vi "EngineTagsUI.vi"() -> ()   [LabVIEW 2013, in "PL Framework Configuration Tool.lvlib" / "EngineTags.lvclass"]
uses:
  EngineTags.lvclass
  <vilib>/NI/Configuration Framework/Node/NodeRef.ctl
  <vilib>/NI/Configuration Framework/Node/NISE_CEF_Node.lvclass
  <vilib>/NI/AMC/Message Queue.ctl
  <vilib>/NI/AMC/Message.ctl
  <vilib>/NI/Tools/Keyed Array/KeyedArray.ctl
  <vilib>/NI/Configuration Framework/Node/UserEventRef.ctl
  <vilib>/NI/Configuration Framework/Controls/EventCluster.ctl
  <vilib>/NI/Tag Bus/tag/Data Type.ctl
  <vilib>/NI/Configuration Framework/Node/RefreshUIEvent.ctl
  <vilib>/NI/Configuration Framework/Node/CacheState.ctl
  <vilib>/NI/Configuration Framework/Node/StopEvent.ctl
  <vilib>/NI/Configuration Framework/Node/NodeChangeEvent.ctl
  additional filter.ctl
  <vilib>/Utility/miscctls.llb/LVPositionTypeDef.ctl
  <vilib>/NI/Module Execution Interface/Engine Configuration/engine configuration.lvclass/engine configuration.ctl
  <vilib>/NI/Tag Bus/tag/tag descriptor.lvclass/tag descriptor.ctl
  <vilib>/NI/Tag Bus/tag/read tag name.vi
  <vilib>/NI/Tag Bus/tag/read data type.vi
  <vilib>/NI/Tag Bus/tag/read raw default value.vi
  <vilib>/NI/Tag Bus/tag/read metadata.vi
  <vilib>/NI/Module Execution Interface/Engine Configuration/engine configuration.lvclass
  Engine Parent/Engine Parent Editor Node.lvclass
  <vilib>/NI/Tag Bus/tag/tag descriptor.lvclass
  <vilib>/NI/Tools/Keyed Array/Tools_KeyedArray.lvlib
  <vilib>/NI/AMC/AMC.lvlib
  <vilib>/NI/Configuration Framework/NISE_CEF_TreeControl.lvlib
panel:
  in  "more filters":T1
  in  "Remove Button":bool
  in  "node change":T2
  in  "stop event":T3
  in  "cache state":T4
  in  "refresh UI":T5
  in  "Filter":string
  in  "export to csv":bool
  in  "open csv":bool
  in  "open cvtv3 taglist":bool
  in  "load CVT1 file":bool
  in  "Create Tag":bool
  in  "data type":T6
  in  "Table":string[][](table)
  in  "user event":T7
  in  "main queue":T8
  in  "node ref":T9
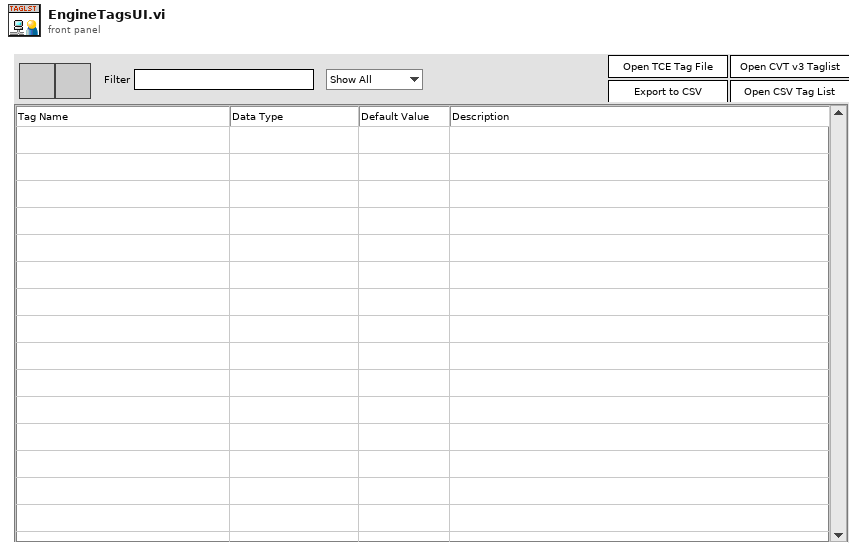
[diagram p1: front panel]
types:
  T1 = typedef "PL Framework Configuration Tool.lvlib/EngineTags.lvclass/additional filter.ctl" = enum16{"Show All", "Show Unmapped"}
  T2 = typedef "NISE_CEF_Node.lvclass/NodeChangeEvent.ctl" = refnum<user-event>
  T3 = typedef "NISE_CEF_Node.lvclass/StopEvent.ctl" = refnum<user-event>
  T4 = typedef "NISE_CEF_Node.lvclass/CacheState.ctl" = refnum<user-event>
  T5 = typedef "NISE_CEF_Node.lvclass/RefreshUIEvent.ctl" = refnum<user-event>
  T6 = typedef "tag bus.lvlib/tag descriptor.lvclass/Data Type.ctl" = enum16{"Double", "Single", "I64", "I32", "I16", "I8", "U64", "U32", "U16", "U8", "Boolean", "String", "Array of Double", "Array of Single", "Array of I64", "Array of I32", "Array of I16", "Array of I8", "Array of U64", "Array of U32", "Array of U16", "Array of U8", "Array of Boolean", "Array of String"}
  T7 = typedef "NISE_CEF_Node.lvclass/UserEventRef.ctl" = refnum<user-event>
  T8 = typedef "AMC.lvlib/Message Queue.ctl" = refnum<queue>
  T9 = typedef "NISE_CEF_Node.lvclass/NodeRef.ctl" = refnum<data-value>
  T10 = typedef "LVPositionTypeDef.ctl" = cluster{"Left":i32, "Top":i32}
  T11 = enum16{"open", "replace", "create", "open or create", "replace or create", "replace or create with confirmation"}
  T12 = typedef "LVPoint32TypeDef.ctl" = cluster{"Horizontal":i32, "Vertical":i32}
  T13 = typedef "LVRowAndColumnTypeDef.ctl" = cluster{"Row":i32, "Column":i32}
  T14 = typedef "LVBoundsTypeDef.ctl" = cluster{"Width":u32, "Height":u32}
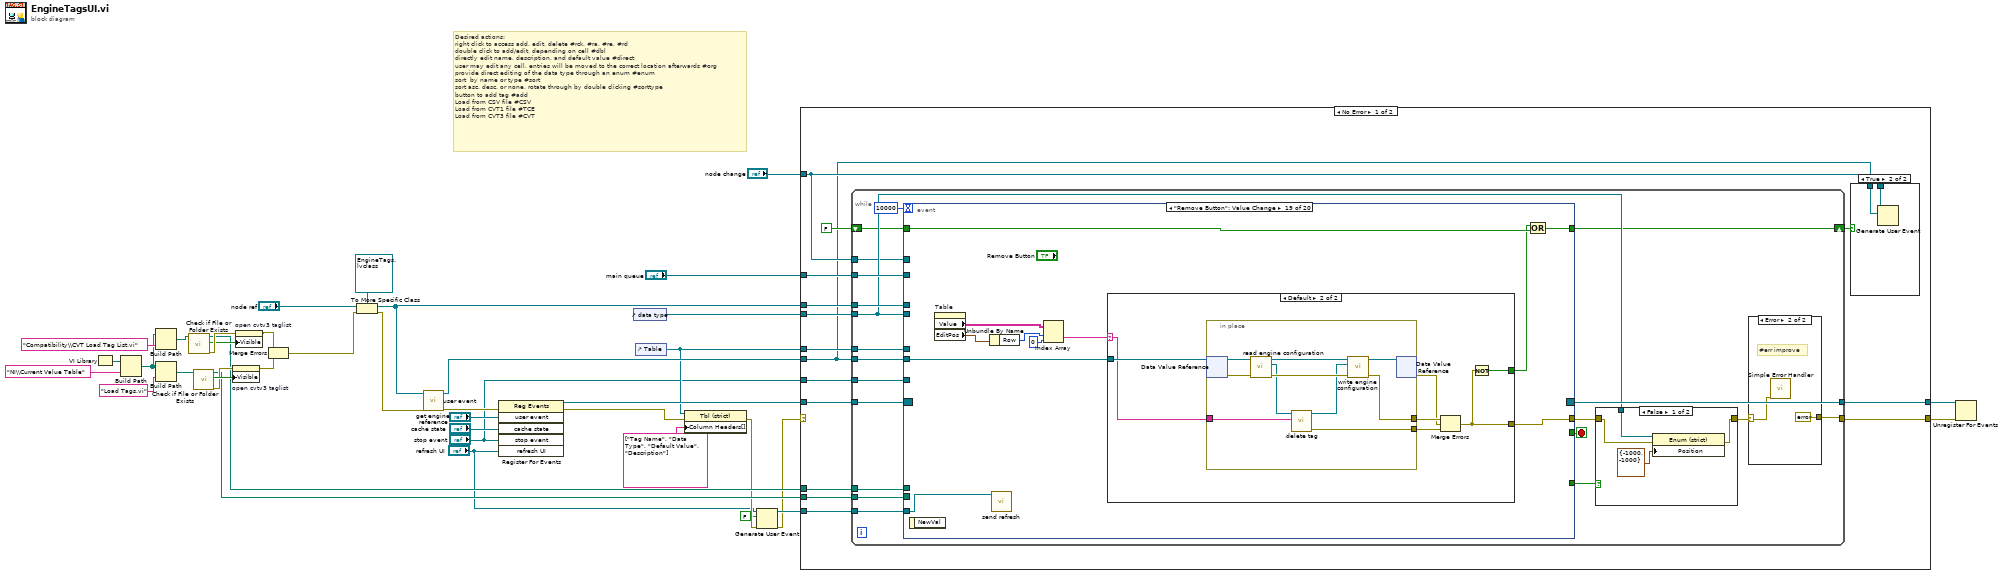
[diagram p0: block diagram]
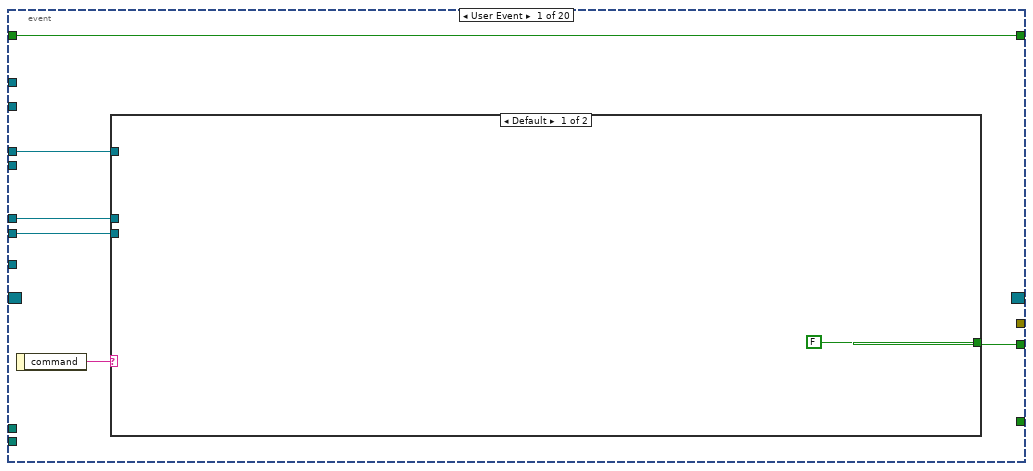
[diagram p5: hidden frame]
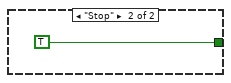
[diagram p6: hidden frame]
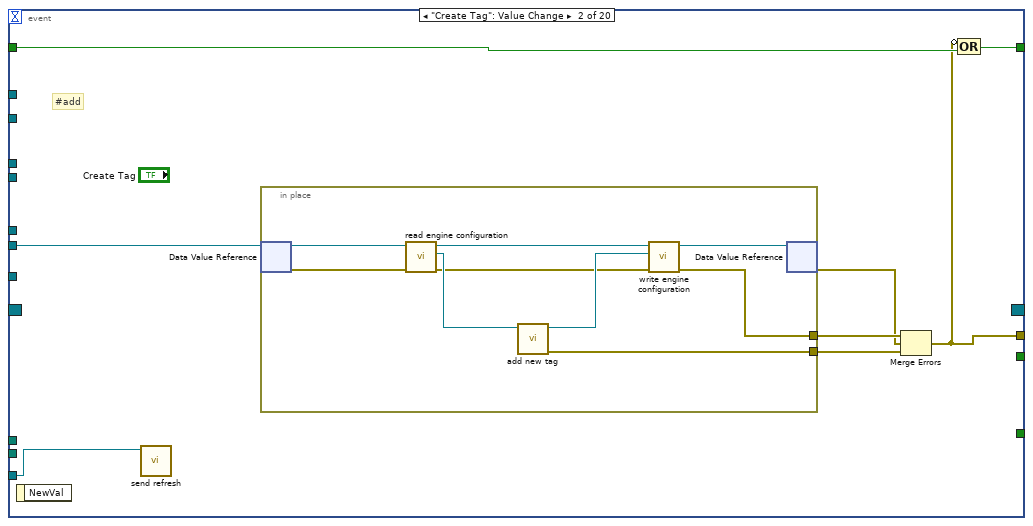
[diagram p7: hidden frame]
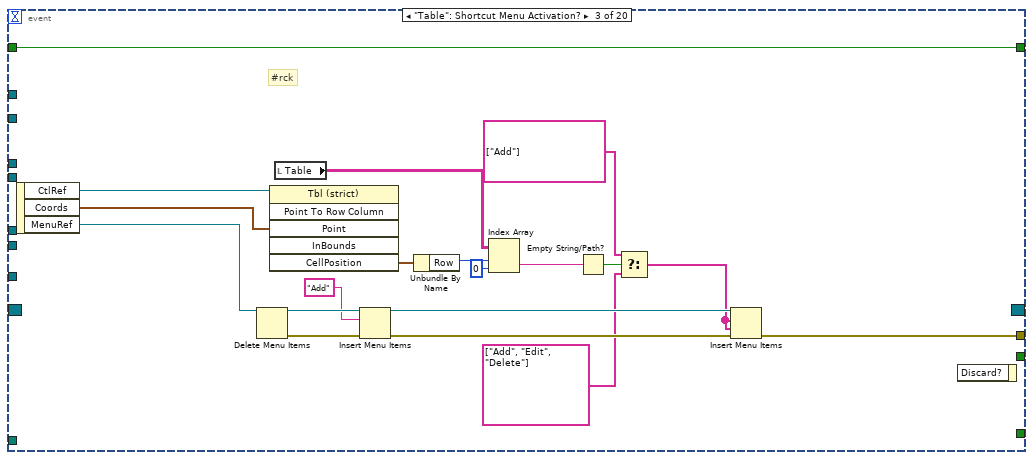
[diagram p8: hidden frame]
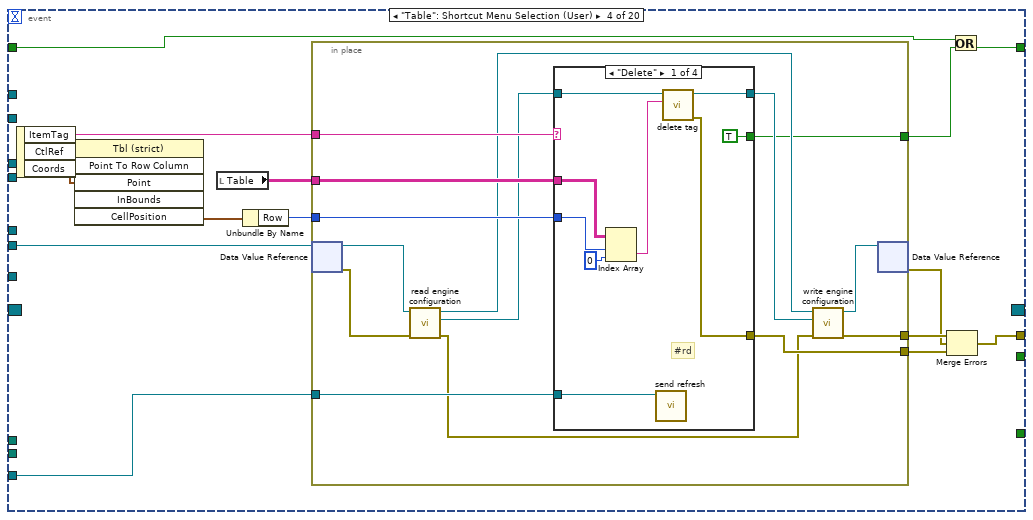
[diagram p9: hidden frame]
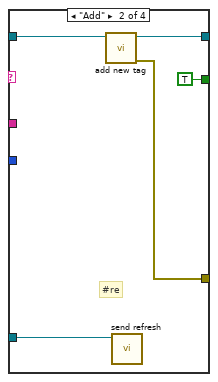
[diagram p10: hidden frame]
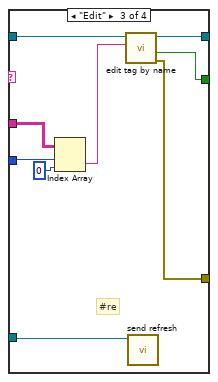
[diagram p11: hidden frame]
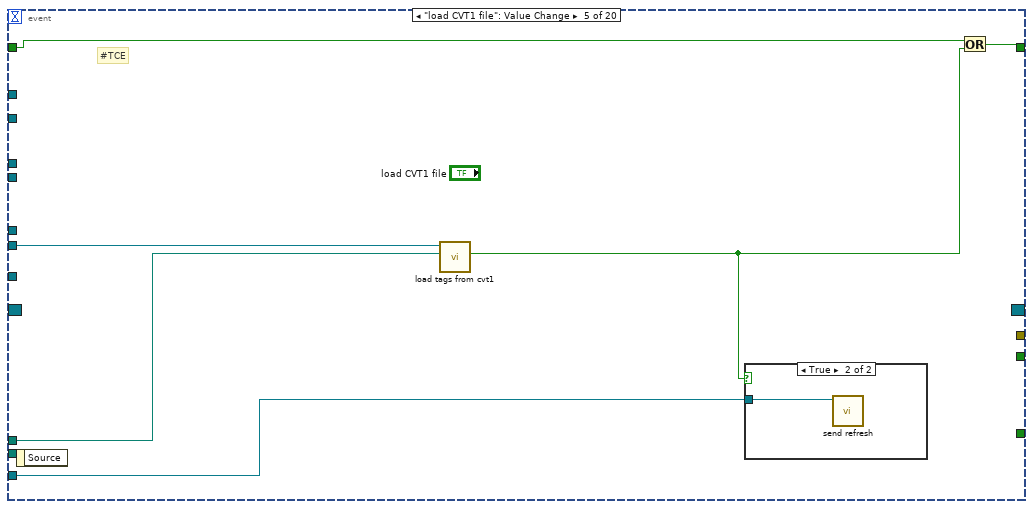
[diagram p13: hidden frame]
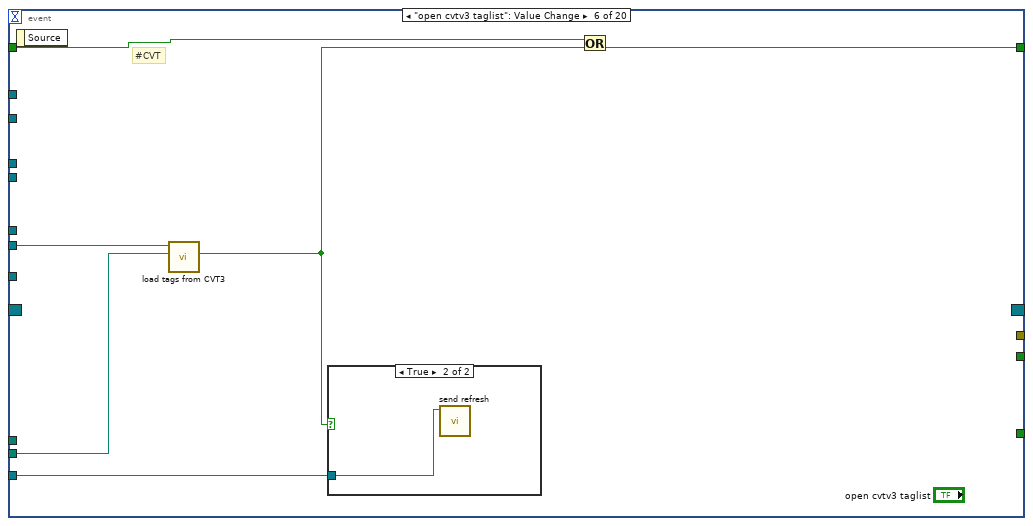
[diagram p15: hidden frame]
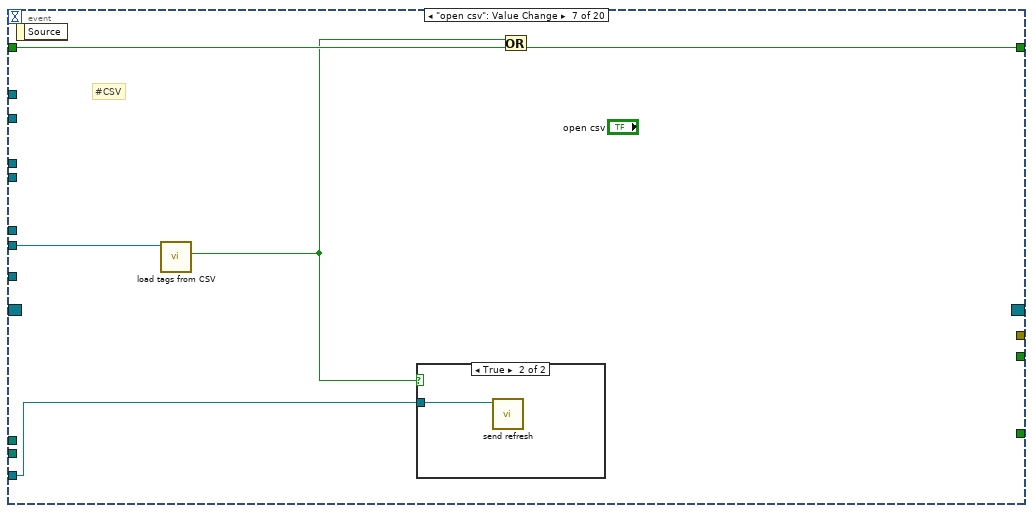
[diagram p17: hidden frame]
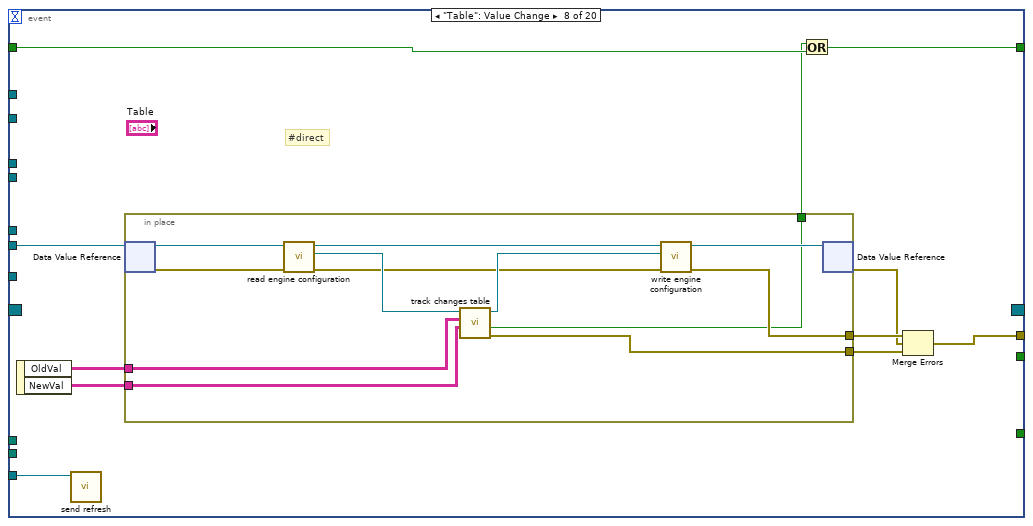
[diagram p19: hidden frame]
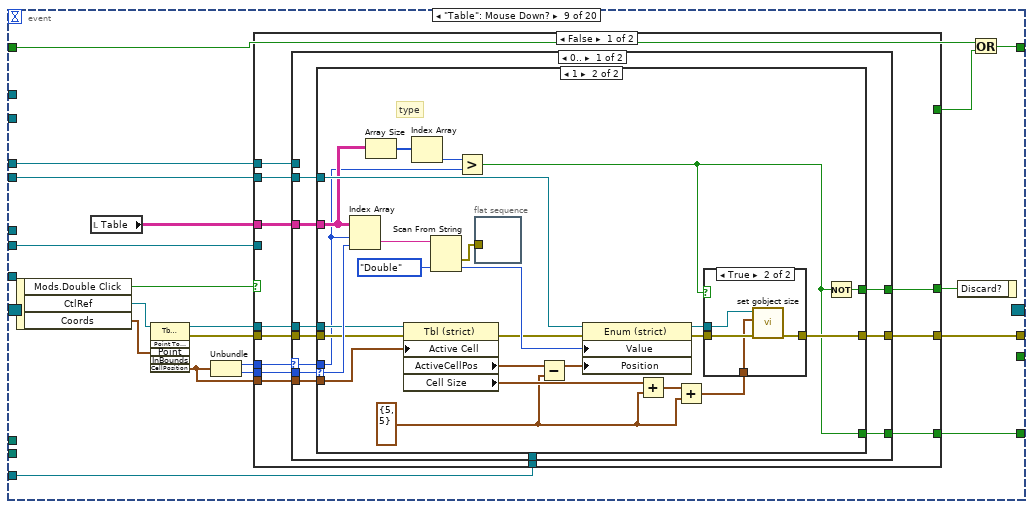
[diagram p20: hidden frame]
diagram:
  # "Desired actions:\nright click to access add, edit, delete #rck, #ra, #re, #rd\ndouble click to add/edit, depending on cell #dbl\ndirectly edit name, description, and default value #direct\nuser may edit any cell, entries will be moved to the correct location afterwards #org\nprovide direct editing of the data type through an enum #enum\nsort  by name or type #sort\nsort asc, desc, or none, rotate through by double clicking #sorttype\nbutton to add tag #add\nLoad from CSV file #CSV\nLoad from CVT1 file #TCE\nLoad from CVT3 file #CVT"
  n1 = VI Library() -> (path=w34:path)
  n2 = Build Path(base path=w34, name or relative path="NI\\Current Value Table") -> (appended path=w30:path)
  n3 = Build Path(base path=w30, name or relative path="Compatibility\\CVT Load Tag List.vi") -> (appended path=w23:path)
  n4 = Build Path(base path=w30, name or relative path="Load Tags.vi") -> (appended path=w21:path)
  n5 = call <vilib>:"Check if File or Folder Exists.vi"("path"=w23) -> ("error out"=w27:errorcluster, "file or folder exists?"=w26:bool, "dup path"=w22:path)  [unwired: 8 in]
  n6 = call <vilib>:"Check if File or Folder Exists.vi"("path"=w21) -> ("error out"=w28:errorcluster, "file or folder exists?"=w29:bool, "dup path"=w20:path)  [unwired: 8 in]
  n7 = property on="open cvtv3 taglist" class="Bool"(error in=w28, "Visible"=w29) -> (error out=w25:errorcluster)  [unwired: 1 in, 1 out]
  n8 = property on="open cvtv3 taglist" class="Bool"(error in=w27, "Visible"=w26) -> (error out=w24:errorcluster)  [unwired: 1 in, 1 out]
  n9 = Merge Errors(w24, w25) -> (w19:errorcluster)
  n10 = To More Specific Class(target class=refnum<data-value> refnum ("data value reference"), reference="node ref", error in=w19) -> (specific class reference=w18:refnum<data-value>, error out=w6:errorcluster)
  n11 = call "get engine reference.vi"("error in"=w6, "enginetags"=w18) -> ("error out"=w15:errorcluster, "engine reference"=w14:refnum<data-value>)  [unwired: 8 in]
  n12 = register-events(error in=w15, "user event", "cache state", "stop event", "refresh UI") -> (reference out=w38:refnum<event-registration>, error out=w35:errorcluster)  [unwired: 1 in]
  n13 = control-ref of="data type"() -> (w16:refnum<vi>)
  n14 = control-ref of="Table"() -> (w13:refnum<vi>)
  n15 = property on="Property Node" class="Tbl (strict)"(reference=w13, error in=w35, "Column Headers[]"=string[] ["Tag Name", "Data Type", "Default Value", "Description"] ("Column Header Strings[]")) -> (error out=w9:errorcluster)  [unwired: 1 out]
  n16 = Generate User Event(user event="refresh UI", event data cluster=FALSE ("event data"), error in=w9) -> (user event out=w10:T5, error out=w8:errorcluster)  [unwired: 1 in]
  n17 = case shown="No Error" w8 {
    selector: w8 -> [_ w514]
    tunnel: "main queue" -> [w54 _]
    tunnel: w38 -> [w53 w515]
    tunnel: [w52 w515] -> w37
    tunnel: [w51 w514] -> w36
    tunnel: w22 -> [w50 _]
    tunnel: w20 -> [w49 _]
    tunnel: w18 -> [w48 _]
    tunnel: w16 -> [w47 _]
    tunnel: w14 -> [w41 _]
    tunnel: w13 -> [w46 _]
    tunnel: w10 -> [w45 _]
    tunnel: "node change" -> [w42 _]
    tunnel: "stop event" -> [w40 _]
    frame No Error {
      n18 = while {
        tunnel: w48 -> [w68]
        tunnel: w54 -> [w76]
        tunnel: w53 -> [w75]
        tunnel: [w74] -> w52
        tunnel: w49 -> [w72]
        tunnel: w50 -> [w71]
        tunnel: w47 -> [w63]
        tunnel: w41 -> [w69]
        tunnel: w46 -> [w67]
        tunnel: w45 -> [w62]
        tunnel: [w70] -> w51
        shift-right: [w58] -> w43
        shift-left: FALSE -> [w59]
        tunnel: w42 -> [w61]
        tunnel: w40 -> [w57]
        stop <- w73 stop-if-true
        n19 = event shown="[18] \"Remove Button\": Value Change" {
          selector: w75 -> [_ _ _ _ _ _ _ _ _ _ _ _ _ _ _ _ w455 _ _ _]
          dyn-events: [_ _ _ _ _ _ _ _ _ _ _ _ _ _ _ _ _ _ _ _] -> w74
          timeout: 10000 -> [_ _ _ _ _ _ _ _ _ _ _ _ _ _ _ _ _ _ _ _]
          tunnel: w68 -> [w87 _ _ _ _ _ _ _ w237 _ _ _ _ _ _ _ w464 _ _ _]
          tunnel: w76 -> [_ _ _ _ _ _ _ _ _ _ _ _ _ _ _ _ _ _ _ _]
          tunnel: [w89 _ _ _ _ _ _ _ _ _ _ _ _ _ _ TRUE FALSE _ _ _] -> w73
          tunnel: w72 -> [_ _ _ _ _ w194 _ _ _ _ _ _ _ _ _ _ _ _ _ _]
          tunnel: w71 -> [_ _ _ _ w187 _ _ _ _ _ _ _ _ _ _ _ _ _ _ _]
          tunnel: [_ w93 w117 w134 _ _ _ w208 w239 w350 w400 w407 _ w440 _ _ w467 _ w488 w510] -> w64
          tunnel: w63 -> [_ _ _ _ _ _ _ _ w233 w369 _ _ _ _ _ _ _ _ _ _]
          tunnel: w69 -> [w90 w99 _ w135 w185 w192 w199 w209 w228 w351 _ w404 _ _ _ _ w466 w475 w492 _]
          tunnel: w67 -> [w86 _ _ _ _ _ _ _ _ w370 _ _ _ _ _ _ w463 _ _ _]
          tunnel: [_ _ _ _ _ _ _ _ w230 _ _ _ _ _ _ _ _ _ _ _] -> w66
          tunnel: w62 -> [_ w95 _ w136 w186 w193 w200 w202 w229 w347 _ _ w437 _ _ _ _ _ w490 w512]
          tunnel: w61 -> [_ _ _ _ _ _ _ _ _ _ _ _ _ _ _ _ _ w476 _ _]
          tunnel: w59 -> [w85 w96 w110 w131 w184 w191 w198 w205 w227 _ w399 w402 w438 w439 w443 w448 w453 w477 w491 w513]
          tunnel: [w85 w94 w110 w130 w183 w190 w197 w204 w226 TRUE w399 w402 w438 w439 w443 w448 w452 w474 w489 w513] -> w58
          tunnel: w57 -> [_ _ _ _ _ _ _ _ _ _ w398 _ _ _ _ _ _ _ _ _]
          event User Event {
            n20 = event-data() -> ("command"=w88:string)  [unwired: 1 in]
            n21 = case shown="Default" w88 {
              tunnel: w90 -> [_ _]
              tunnel: [FALSE TRUE] -> w89
              tunnel: w87 -> [_ _]
              tunnel: w86 -> [_ _]
              frame Default {
              }
              frame "Stop" {
              }
            }
          }
          event "Create Tag": Value Change {
            # "#add"
            n22 = event-data() -> ()  [unwired: 1 in, 1 out]
            n23 = call "send refresh.vi"("refresh UI"=w95) -> ()  [unwired: 11 in]
            n24 = in-place {
              in-place-border: [w109] -> w100
              in-place-border: [w102] -> w97
              n25 = in-place-dvr #1(w99) -> (w104:refnum<class "Engine Parent Editor Node.lvclass">, w105:errorcluster)
              n26 = call "read engine configuration.vi"("error in"=w105, "Engine Parent Editor Node in"=w104) -> ("error out"=w101:errorcluster, "engine configuration"=w108:refnum<class "engine configuration.lvclass">, "Engine Parent Editor Node out"=w106:refnum<class "Engine Parent Editor Node.lvclass">)  [unwired: 7 in]
              n27 = call "add new tag.vi"("engine configuration in"=w108) -> ("error out"=w102:errorcluster, "engine configuration out"=w107:refnum<class "engine configuration.lvclass">)  [unwired: 9 in]
              n28 = call "write engine configuration.vi"("error in"=w101, "engine configuration"=w107, "Engine Parent Editor Node in"=w106) -> ("error out"=w109:errorcluster, "Engine Parent Editor Node out"=w103:refnum<class "Engine Parent Editor Node.lvclass">)  [unwired: 7 in]
              n29 = in-place-dvr #1(w103) -> (w98:errorcluster)  [unwired: 1 out]
            }
            n30 = Merge Errors(w100, w98, w97) -> (w93:errorcluster)
            n31 = Compound Arithmetic op=OR(invert w93, w96) -> (w94:bool)
          }
          event "Table": Shortcut Menu Activation? {
            # "#rck"
            n32 = event-data() -> ("CtlRef"=w123:refnum<vi>, "Coords"=w124:T12, "MenuRef"=w122:refnum<k9>)  [unwired: 1 in]
            n33 = Delete Menu Items(9:w122) -> (0:w127:errorcluster, 3:w128:refnum<k9>)  [unwired: 3 in]
            n34 = invoke class="Tbl (strict)" method="Point To Row Column"(reference=w123, "Point"=w124) -> ("CellPosition"=w125:T13)  [unwired: 4 in, 5 out]
            n35 = local read "Table"() -> (w121:string[][])
            n36 = Insert Menu Items(6:w127, 8:"Add", 9:w128) -> (0:w116:errorcluster, 3:w118:refnum<k9>)  [unwired: 3 in, 1 out]
            n37 = Unbundle By Name(w125) -> ("Row"=w120:i32)
            n38 = Index Array(array=w121, index (row)=w120, index (col)=0 ("disabled index (col)")) -> (element=w115:string)
            n39 = Empty String/Path?(string/path=w115) -> (empty?=w114:bool)
            n40 = Select(t=string[] ["Add"], s=w114, f=string[] ["Add", "Edit", "Delete"]) -> (s? t:f=w111:string[])
            n41 = Insert Menu Items(6:w116, 7:w111, 8:w111, 9:w118) -> (0:w117:errorcluster)  [unwired: 2 in, 2 out]
            n42 = event-data() -> ()  [unwired: 2 in, 1 out]
          }
          event "Table": Shortcut Menu Selection (User) {
            n43 = event-data() -> ("ItemTag"=w143:string, "CtlRef"=w142:refnum<vi>, "Coords"=w141:T12)  [unwired: 1 in]
            n44 = invoke class="Tbl (strict)" method="Point To Row Column"(reference=w142, "Point"=w141) -> ("CellPosition"=w140:T13)  [unwired: 4 in, 5 out]
            n45 = local read "Table"() -> (w137:string[][])
            n46 = Unbundle By Name(w140) -> ("Row"=w139:i32)
            n47 = in-place {
              in-place-border: w143 -> [w157]
              in-place-border: w139 -> [w156]
              in-place-border: [w151] -> w138
              in-place-border: w137 -> [w155]
              in-place-border: w136 -> [w154]
              in-place-border: [w146] -> w132
              in-place-border: [w144] -> w129
              n48 = in-place-dvr #2(w135) -> (w152:refnum<class "Engine Parent Editor Node.lvclass">, w153:errorcluster)
              n49 = call "read engine configuration.vi"("error in"=w153, "Engine Parent Editor Node in"=w152) -> ("error out"=w145:errorcluster, "engine configuration"=w148:refnum<class "engine configuration.lvclass">, "Engine Parent Editor Node out"=w149:refnum<class "Engine Parent Editor Node.lvclass">)  [unwired: 7 in]
              n50 = case shown="\"Delete\"" w157 {
                tunnel: w156 -> [w165 _ w179 _]
                tunnel: [w163 w170 w176 w181] -> w147
                tunnel: w148 -> [w164 w171 w177 w181]
                tunnel: [w160 w169 w174 _] -> w146
                tunnel: w155 -> [w161 _ w175 _]
                tunnel: w154 -> [w159 w168 w173 _]
                tunnel: [TRUE TRUE w172 _] -> w144
                frame "Delete" {
                  # "#rd"
                  n51 = Index Array(array=w161, index (row)=w165, index (col)=0 ("disabled index (col)")) -> (element=w162:string)
                  n52 = call "send refresh.vi"("refresh UI"=w159) -> ()  [unwired: 11 in]
                  n53 = call <vilib>:"delete tag.vi"("tag name"=w162, "engine configuration in"=w164) -> ("error out"=w160:errorcluster, "engine configuration out"=w163:refnum<class "engine configuration.lvclass">)  [unwired: 8 in]
                }
                frame "Add" {
                  # "#re"
                  n54 = call "add new tag.vi"("engine configuration in"=w171) -> ("error out"=w169:errorcluster, "engine configuration out"=w170:refnum<class "engine configuration.lvclass">)  [unwired: 9 in]
                  n55 = call "send refresh.vi"("refresh UI"=w168) -> ()  [unwired: 11 in]
                }
                frame "Edit" {
                  # "#re"
                  n56 = Index Array(array=w175, index (row)=w179, index (col)=0 ("disabled index (col)")) -> (element=w178:string)
                  n57 = call "edit tag by name.vi"("name"=w178, "engine configuration in"=w177) -> ("error out"=w174:errorcluster, "change?"=w172:bool, "engine configuration out"=w176:refnum<class "engine configuration.lvclass">)  [unwired: 7 in]
                  n58 = call "send refresh.vi"("refresh UI"=w173) -> ()  [unwired: 11 in]
                }
                frame Default {
                }
              }
              n59 = call "write engine configuration.vi"("error in"=w145, "engine configuration"=w147, "Engine Parent Editor Node in"=w149) -> ("error out"=w151:errorcluster, "Engine Parent Editor Node out"=w150:refnum<class "Engine Parent Editor Node.lvclass">)  [unwired: 7 in]
              n60 = in-place-dvr #2(w150) -> (w133:errorcluster)  [unwired: 1 out]
            }
            n61 = Merge Errors(w138, w133, w132) -> (w134:errorcluster)
            n62 = Or(x=w131, y=w129) -> (x .or. y?=w130:bool)
          }
          event "load CVT1 file": Value Change {
            # "#TCE"
            n63 = event-data() -> ()  [unwired: 1 in, 1 out]
            n64 = call "load tags from cvt1.vi"("vi path"=w187, "engine ref"=w185) -> ("load attempted"=w182:bool)  [unwired: 9 in]
            n65 = case shown="True" w182 {
              tunnel: w186 -> [_ w188]
              frame False {
              }
              frame True {
                n66 = call "send refresh.vi"("refresh UI"=w188) -> ()  [unwired: 11 in]
              }
            }
            n67 = Or(x=w184, y=w182) -> (x .or. y?=w183:bool)
          }
          event "open cvtv3 taglist": Value Change {
            # "#CVT"
            n68 = event-data() -> ()  [unwired: 1 in, 1 out]
            n69 = call "load tags from CVT3.vi"("path"=w194, "engine ref"=w192) -> ("load attempted"=w189:bool)  [unwired: 9 in]
            n70 = case shown="True" w189 {
              tunnel: w193 -> [_ w195]
              frame False {
              }
              frame True {
                n71 = call "send refresh.vi"("refresh UI"=w195) -> ()  [unwired: 11 in]
              }
            }
            n72 = Or(x=w191, y=w189) -> (x .or. y?=w190:bool)
          }
          event "open csv": Value Change {
            # "#CSV"
            n73 = event-data() -> ()  [unwired: 1 in, 1 out]
            n74 = call "load tags from CSV.vi"("engine ref"=w199) -> ("load attempted"=w196:bool)  [unwired: 10 in]
            n75 = case shown="True" w196 {
              tunnel: w200 -> [_ w201]
              frame False {
              }
              frame True {
                n76 = call "send refresh.vi"("refresh UI"=w201) -> ()  [unwired: 11 in]
              }
            }
            n77 = Or(x=w196, y=w198) -> (x .or. y?=w197:bool)
          }
          event "Table": Value Change {
            # "#direct"
            n78 = event-data() -> ("OldVal"=w211:string[][], "NewVal"=w212:string[][])  [unwired: 1 in]
            n79 = call "send refresh.vi"("refresh UI"=w202) -> ()  [unwired: 11 in]
            n80 = in-place {
              in-place-border: w212 -> [w224]
              in-place-border: w211 -> [w223]
              in-place-border: [w221] -> w210
              in-place-border: [w214] -> w206
              in-place-border: [w213] -> w203
              n81 = in-place-dvr #3(w209) -> (w219:refnum<class "Engine Parent Editor Node.lvclass">, w222:errorcluster)
              n82 = call "read engine configuration.vi"("error in"=w222, "Engine Parent Editor Node in"=w219) -> ("error out"=w215:errorcluster, "engine configuration"=w216:refnum<class "engine configuration.lvclass">, "Engine Parent Editor Node out"=w220:refnum<class "Engine Parent Editor Node.lvclass">)  [unwired: 7 in]
              n83 = call "track changes table.vi"("NewVal"=w224, "OldVal"=w223, "Engine Input"=w216) -> ("error out"=w214:errorcluster, "change?"=w213:bool, "Engine Output"=w217:refnum<class "engine configuration.lvclass">)  [unwired: 6 in]
              n84 = call "write engine configuration.vi"("error in"=w215, "engine configuration"=w217, "Engine Parent Editor Node in"=w220) -> ("error out"=w221:errorcluster, "Engine Parent Editor Node out"=w218:refnum<class "Engine Parent Editor Node.lvclass">)  [unwired: 7 in]
              n85 = in-place-dvr #3(w218) -> (w207:errorcluster)  [unwired: 1 out]
            }
            n86 = Or(x=w203, y=w205) -> (x .or. y?=w204:bool)
            n87 = Merge Errors(w210, w207, w206) -> (w208:errorcluster)
          }
          event "Table": Mouse Down? {
            n88 = event-data() -> ("Mods.Double Click"=w241:bool, "CtlRef"=w243:refnum<vi>, "Coords"=w242:T12)  [unwired: 1 in]
            n89 = local read "Table"() -> (w236:string[][])
            n90 = invoke class="Tbl (strict)" method="Point To Row Column"(reference=w243, "Point"=w242) -> (reference out=w232:refnum<vi>, error out=w240:errorcluster, "CellPosition"=w231:T13)  [unwired: 4 in, 3 out]
            n91 = Unbundle(w231) -> ("Row"=w235:i32, "Column"=w234:i32)
            n92 = case shown="False" w241 {
              tunnel: w240 -> [w252 w307]
              tunnel: [w253 w306] -> w239
              tunnel: [w254 TRUE] -> w238
              tunnel: w237 -> [w250 w308]
              tunnel: w236 -> [w248 w305]
              tunnel: w235 -> [w255 w304]
              tunnel: w234 -> [w251 w303]
              tunnel: w233 -> [w249 _]
              tunnel: w232 -> [w247 _]
              tunnel: w231 -> [w246 _]
              tunnel: [w245 _] -> w230
              tunnel: w229 -> [w244 w300]
              tunnel: w228 -> [_ w302]
              tunnel: [_ w301] -> w225
              frame False {
                n93 = case shown="0.." w255 {
                  selector: w255 -> [w259 _]
                  tunnel: [w264 FALSE] -> w254
                  tunnel: [w262 w298] -> w253
                  tunnel: w252 -> [w263 w298]
                  tunnel: w251 -> [w265 _]
                  tunnel: w250 -> [_ _]
                  tunnel: w249 -> [w261 _]
                  tunnel: w248 -> [w260 _]
                  tunnel: w247 -> [w258 _]
                  tunnel: w246 -> [w257 _]
                  tunnel: [w256 _] -> w245
                  tunnel: w244 -> [_ _]
                  frame 0.. {
                    n94 = case shown="1" w265 {
                      selector: w265 -> [_ w292]
                      tunnel: [FALSE w268] -> w264
                      tunnel: w263 -> [w266 w283]
                      tunnel: [w266 w286] -> w262
                      tunnel: w261 -> [_ w288]
                      tunnel: w260 -> [_ w273]
                      tunnel: w259 -> [_ w270]
                      tunnel: w258 -> [_ w282]
                      tunnel: w257 -> [_ w281]
                      tunnel: [_ w269] -> w256
                      frame Default {
                        # "any other column, direct edit"
                      }
                      frame 1 {
                        w274 = T10 {"Left"=5, "Top"=5} ("Active Cell:Position")
                        # "type"
                        n95 = Index Array(array=w273, index (row)=w270, index (col)=w292) -> (element=w291:string)
                        n96 = Array Size(array=w273) -> (size(s)=w272:i32[])
                        n97 = property on="Property Node" class="Tbl (strict)"(reference=w282, error in=w283, "Active Cell"=w281) -> (error out=w279:errorcluster, "ActiveCellPos"=w280:T10, "Cell Size"=w278:T14)  [unwired: 1 out]
                        n98 = Index Array(array=w272) -> (element=w271:i32)  [unwired: 1 in]
                        n99 = Scan From String(input string=w291, default 1=Data_Type."Double" ("Value")) -> (error out=w289:errorcluster, output 1=w284:T6)  [unwired: 3 in, 2 out]
                        n100 = Greater?(x=w271, y=w270) -> (0:w269:bool)
                        n101 = flat-sequence {
                          tunnel: w289 -> [_]
                          frame #0 {
                          }
                        }
                        n102 = Subtract(x=w280, y=w274) -> (x-y=w275:T10)
                        n103 = property on="Property Node" class="Enum (strict)"(reference=w288, error in=w279, "Value"=w284, "Position"=w275) -> (reference out=w285:refnum<vi>, error out=w287:errorcluster)
                        n104 = Add(x=w278, y=w274) -> (x+y=w277:T14)
                        n105 = Add(x=w277, y=w274) -> (x+y=w276:T14)
                        n106 = case shown="True" w269 {
                          tunnel: w287 -> [w293 w297]
                          tunnel: [w293 w296] -> w286
                          tunnel: w285 -> [_ w295]
                          tunnel: w276 -> [_ w294]
                          frame False {
                          }
                          frame True {
                            n107 = call "set gobject size.vi"("error in"=w297, "size"=w294, "object refnum"=w295) -> ("error out"=w296:errorcluster)  [unwired: 8 in]
                          }
                        }
                        n108 = Not(x=w269) -> (.not. x?=w268:bool)
                      }
                    }
                  }
                  frame ..-1 {
                    # "header"
                  }
                }
              }
              frame True {
                n109 = case shown="0.." w304 {
                  selector: w304 -> [w319 _]
                  tunnel: w303 -> [_ w342]
                  tunnel: w308 -> [_ w345]
                  tunnel: w307 -> [w318 w344]
                  tunnel: [w313 w343] -> w306
                  tunnel: w305 -> [w320 _]
                  tunnel: w302 -> [w314 _]
                  tunnel: [TRUE _] -> w301
                  frame 0.. {
                    # "#dbl"
                    n110 = Index Array(array=w320, index (row)=w319, index (col)=0 ("disabled index (col)")) -> (element=w317:string)
                    n111 = in-place {
                      in-place-border: w318 -> [w332]
                      in-place-border: w317 -> [w331]
                      in-place-border: [w330] -> w316
                      in-place-border: [w324] -> w311
                      n112 = in-place-dvr #4(w314) -> (w326:refnum<class "Engine Parent Editor Node.lvclass">, w323:errorcluster)
                      n113 = Merge Errors(w332, w323) -> (w322:errorcluster)
                      n114 = call "read engine configuration.vi"("error in"=w323, "Engine Parent Editor Node in"=w326) -> ("error out"=w321:errorcluster, "engine configuration"=w329:refnum<class "engine configuration.lvclass">, "Engine Parent Editor Node out"=w327:refnum<class "Engine Parent Editor Node.lvclass">)  [unwired: 7 in]
                      n115 = case shown="\"\"" w331 {
                        selector: w331 -> [w334 _]
                        tunnel: w322 -> [w333 w338]
                        tunnel: w329 -> [w337 w341]
                        tunnel: [w336 w340] -> w325
                        tunnel: [w335 w339] -> w324
                        frame Default {
                          n116 = call "edit tag by name.vi"("error in"=w333, "name"=w334, "engine configuration in"=w337) -> ("error out"=w335:errorcluster, "engine configuration out"=w336:refnum<class "engine configuration.lvclass">)  [unwired: 6 in, 1 out]
                        }
                        frame "" {
                          n117 = call "add new tag.vi"("error in"=w338, "engine configuration in"=w341) -> ("error out"=w339:errorcluster, "engine configuration out"=w340:refnum<class "engine configuration.lvclass">)  [unwired: 8 in]
                        }
                      }
                      n118 = call "write engine configuration.vi"("error in"=w321, "engine configuration"=w325, "Engine Parent Editor Node in"=w327) -> ("error out"=w330:errorcluster, "Engine Parent Editor Node out"=w328:refnum<class "Engine Parent Editor Node.lvclass">)  [unwired: 7 in]
                      n119 = in-place-dvr #4(w328) -> (w312:errorcluster)  [unwired: 1 out]
                    }
                    n120 = Merge Errors(w316, w312, w311) -> (w313:errorcluster)
                  }
                  frame ..-1 {
                    # "clicked on header, rotate through sort options"
                    n121 = call "rotate sorting options.vi"("error in"=w344, "Column"=w342, "taglist"=w345) -> ("error out"=w343:errorcluster)  [unwired: 8 in]
                  }
                }
                n122 = call "send refresh.vi"("refresh UI"=w300) -> ()  [unwired: 11 in]
              }
            }
            n123 = event-data("Discard?"=w238) -> ()  [unwired: 1 in, 1 out]
            n124 = Or(x=w227, y=w225) -> (x .or. y?=w226:bool)
          }
          event Value Change {
            # "#enum"
            n125 = event-data() -> ()  [unwired: 1 in, 1 out]
            n126 = property class="Enum (strict)"(reference=w369) -> (error out=w357:errorcluster, "Left"=w365:i32, "Width"=w368:u32, "Top"=w362:i32, "Height"=w361:u32)  [unwired: 1 in, 1 out]
            n127 = Scale By Power Of 2(n=i16 -1, x=w368) -> (x*2^n=w366:u32)
            n128 = Scale By Power Of 2(n=i16 -1, x=w361) -> (x*2^n=w364:u32)
            n129 = Add(x=w365, y=w366) -> (x+y=w359:u32)
            n130 = Add(x=w362, y=w364) -> (x+y=w360:u32)
            n131 = Bundle(w359, w360) -> (w358:cluster{u32, u32})  [unwired: 1 in]
            n132 = invoke class="Tbl (strict)" method="Point To Row Column"(reference=w370, error in=w357, "Point"=w358) -> (error out=w354:errorcluster, "CellPosition"=w356:T13)  [unwired: 3 in, 4 out]
            n133 = local read "Table"() -> (w371:string[][])
            n134 = Unbundle By Name(w356) -> ("Row"=w355:i32)
            n135 = call "send refresh.vi"("refresh UI"=w347) -> ()  [unwired: 11 in]
            n136 = Index Array(array=w371, index (row)=w355, index (col)=0 ("disabled index (col)")) -> (element=w353:string)
            n137 = in-place {
              in-place-border: "data type" -> [w386]
              in-place-border: w354 -> [w385]
              in-place-border: w353 -> [w384]
              in-place-border: [w379] -> w352
              in-place-border: [w374] -> w348
              n138 = in-place-dvr #5(w351) -> (w382:refnum<class "Engine Parent Editor Node.lvclass">, w383:errorcluster)
              n139 = call "read engine configuration.vi"("error in"=w383, "Engine Parent Editor Node in"=w382) -> ("error out"=w375:errorcluster, "engine configuration"=w376:refnum<class "engine configuration.lvclass">, "Engine Parent Editor Node out"=w381:refnum<class "Engine Parent Editor Node.lvclass">)  [unwired: 7 in]
              n140 = Merge Errors(w385, w375) -> (w378:errorcluster)
              n141 = case shown="\"\"" w384 {
                selector: w384 -> [_ w392]
                tunnel: [w388 w396] -> w377
                tunnel: w386 -> [_ w395]
                tunnel: w378 -> [w390 w394]
                tunnel: [w389 w393] -> w374
                tunnel: w376 -> [w387 w391]
                frame "" {
                  n142 = call "add new tag.vi"("error in"=w390, "engine configuration in"=w387) -> ("error out"=w389:errorcluster, "engine configuration out"=w388:refnum<class "engine configuration.lvclass">)  [unwired: 8 in]
                }
                frame Default {
                  n143 = call <vilib>:"change tag type.vi"("error in"=w394, "new data type"=w395, "tag name"=w392, "engine configuration in"=w391) -> ("error out"=w393:errorcluster, "engine configuration out"=w396:refnum<class "engine configuration.lvclass">)  [unwired: 6 in]
                }
              }
              n144 = call "write engine configuration.vi"("error in"=w375, "engine configuration"=w377, "Engine Parent Editor Node in"=w381) -> ("error out"=w379:errorcluster, "Engine Parent Editor Node out"=w380:refnum<class "Engine Parent Editor Node.lvclass">)  [unwired: 7 in]
              n145 = in-place-dvr #5(w380) -> (w349:errorcluster)  [unwired: 1 out]
            }
            n146 = Merge Errors(w352, w349, w348) -> (w350:errorcluster)
          }
          event Panel Close? {
            n147 = event-data() -> ()  [unwired: 1 in, 4 out]
            n148 = Generate User Event(user event=w398, event data cluster=TRUE ("event data")) -> (error out=w400:errorcluster)  [unwired: 2 in, 1 out]
            n149 = event-data("Discard?"=TRUE) -> ()  [unwired: 1 in, 1 out]
          }
          event "export to csv": Value Change {
            n150 = event-data() -> ()  [unwired: 1 in, 1 out]
            n151 = property class="Engine Parent Editor Node.lvcla"(reference=w404) -> (error out=w405:errorcluster, "Data Access:Engine Configuration"=w403:refnum<class "engine configuration.lvclass">)  [unwired: 1 in, 1 out]
            n152 = call "File Dialog"("pattern (all files)"="*.csv") -> ("selected path"=w408:path, "cancelled"=w412:bool, "error out"=w411:errorcluster)  [unwired: 11 in, 1 out]
            n153 = call <vilib>:"get full tag list.vi"("engine configuration in"=w403) -> ("tag list"=w406:refnum<class "tag descriptor.lvclass">[])  [unwired: 9 in, 1 out]
            n154 = Compound Arithmetic op=AND(invert w412, invert w411) -> (w409:bool)
            n155 = case shown="True" w409 {
              tunnel: w408 -> [_ w423]
              tunnel: [w413 w422] -> w407
              tunnel: w405 -> [w413 w425]
              tunnel: w406 -> [_ w414]
              frame False {
              }
              frame True {
                n156 = Open/Create/Replace File(file path (use dialog)=w423, error in=w425, operation (0:open)=T11."replace or create") -> (refnum out=w421:refnum<file>, error out=w420:errorcluster)  [unwired: 3 in, 1 out]
                n157 = Write to Text File(file (use dialog)=w421, text="Name, Type, Default, Description\n", error in=w420) -> (refnum out=w416:refnum<file>, error out=w418:errorcluster)  [unwired: 1 in, 1 out]
                n158 = for {
                  shift-right: [w436] -> w417
                  shift-left: w418 -> [w432]
                  shift-right: [w434] -> w415
                  shift-left: w416 -> [w435]
                  tunnel: w414 -> [w433] mode=indexing
                  n159 = property class="tag descriptor"(reference=w433, error in=w432) -> (error out=w431:errorcluster, "accessors:name"=w430:string, "accessors:data type"=w429:T6, "accessors:unformatted default"=w428:string, "accessors:metadata"=w427:string)  [unwired: 1 out]
                  n160 = Format Into String(format string="%s,%s,\"%s\",\"%s\"\n", initial string=w435, error in=w431, w430, w429, w428, w427) -> (resulting string=w434:refnum<file>, error out=w436:errorcluster)
                }
                n161 = Close File(refnum=w415, error in=w417) -> (error out=w422:errorcluster)  [unwired: 1 out]
              }
            }
          }
          event "Filter": Value Change {
            n162 = event-data() -> ()  [unwired: 1 in, 6 out]
            n163 = call "send refresh.vi"("refresh UI"=w437) -> ()  [unwired: 11 in]
          }
          event "Filter": Shortcut Menu Activation? {
            w441 = string[] ["Clear"] ("item names")
            n164 = event-data() -> ("MenuRef"=w442:refnum<k9>)  [unwired: 1 in]
            n165 = Insert Menu Items(7:w441, 8:w441, 9:w442) -> (0:w440:errorcluster)  [unwired: 3 in, 2 out]
            n166 = event-data() -> ()  [unwired: 2 in, 1 out]
          }
          event "Filter": Shortcut Menu Selection (User) {
            n167 = event-data() -> ("ItemTag"=w446:string)  [unwired: 1 in]
            n168 = Equal?(x=w446, y="Clear") -> (x = y?=w444:bool)
            n169 = case shown="True" w444 {
              frame False {
              }
              frame True {
                n170 = property on="Filter" class="Str"("Val(Sgnl)"="") -> ()  [unwired: 2 in, 2 out]
              }
            }
          }
          event User Event {
            n171 = event-data() -> ()  [unwired: 1 in, 1 out]
          }
          event User Event {
            n172 = event-data() -> ("UsrEvtRef"=w454:refnum<user-event>)  [unwired: 1 in]
            n173 = Flush Event Queue(0:w455, 2:w454) -> ()  [unwired: 4 in, 3 out]
            n174 = in-place {
              in-place-border: [w473] -> w459
              in-place-border: [w471] -> w451
              n175 = in-place-dvr #6(w466) -> (w469:refnum<class "Engine Parent Editor Node.lvclass">, w473:errorcluster)
              n176 = call "remove mappings to missing channels.vi"("error in"=w473, "Engine Parent Editor Node in"=w469) -> ("error out"=w472:errorcluster, "Engine Parent Editor Node out"=w470:refnum<class "Engine Parent Editor Node.lvclass">)  [unwired: 8 in]
              n177 = Not Equal?(x=w470, y=w469) -> (x != y?=w468:bool)
              n178 = Compound Arithmetic op=AND(w468, invert w472) -> (w471:bool)
              n179 = in-place-dvr #6(w470) -> (w460:refnum<data-value>, w458:errorcluster)
            }
            n180 = Merge Errors(w459, w458) -> (w457:errorcluster)
            n181 = property class="Engine Parent Editor Node.lvcla"(reference=w460, error in=w457) -> (error out=w461:errorcluster, "Data Access:Engine Configuration"=w462:refnum<class "engine configuration.lvclass">)  [unwired: 1 out]
            n182 = Or(x=w453, y=w451) -> (x .or. y?=w452:bool)
            n183 = call "refresh table.vi"("more filters"="more filters", "Filter"="Filter", "error in"=w461, "Table"=w463, "taglist"=w464, "engine configuration in"=w462) -> ("error out"=w467:errorcluster)  [unwired: 5 in]
          }
          event Timeout {
            n184 = event-data() -> ()  [unwired: 1 in, 3 out]
            n185 = case shown="False" w477 {
              selector: w477 -> [w478 _]
              tunnel: w476 -> [_ w481]
              tunnel: w475 -> [_ w480]
              tunnel: [w478 FALSE] -> w474
              frame False {
              }
              frame True {
                n186 = Generate User Event(user event=w481, event data cluster=w480) -> ()  [unwired: 2 in, 2 out]
              }
            }
          }
          event "Remove Button": Value Change {
            n187 = event-data() -> ()  [unwired: 1 in, 1 out]
            n188 = property on="Table" class="Tbl (strict)"() -> ("Value"=w484:string[][], "EditPos"=w487:T13)  [unwired: 2 in, 2 out]
            n189 = Unbundle By Name(w487) -> ("Row"=w485:i32)
            n190 = call "send refresh.vi"("refresh UI"=w490) -> ()  [unwired: 11 in]
            n191 = Index Array(array=w484, index (row)=w485, index (col)=0 ("disabled index (col)")) -> (element=w482:string)
            n192 = case shown="Default" w482 {
              selector: w482 -> [_ w493]
              tunnel: w492 -> [_ w498]
              tunnel: [_ w495] -> w488
              tunnel: [_ w494] -> w483
              frame "" {
              }
              frame Default {
                n193 = in-place {
                  in-place-border: [w509] -> w499
                  in-place-border: [w501] -> w496
                  in-place-border: w493 -> [w500]
                  n194 = in-place-dvr #7(w498) -> (w506:refnum<class "Engine Parent Editor Node.lvclass">, w507:errorcluster)
                  n195 = call "read engine configuration.vi"("error in"=w507, "Engine Parent Editor Node in"=w506) -> ("error out"=w504:errorcluster, "engine configuration"=w503:refnum<class "engine configuration.lvclass">, "Engine Parent Editor Node out"=w508:refnum<class "Engine Parent Editor Node.lvclass">)  [unwired: 7 in]
                  n196 = call <vilib>:"delete tag.vi"("tag name"=w500, "engine configuration in"=w503) -> ("error out"=w501:errorcluster, "engine configuration out"=w502:refnum<class "engine configuration.lvclass">)  [unwired: 8 in]
                  n197 = call "write engine configuration.vi"("error in"=w504, "engine configuration"=w502, "Engine Parent Editor Node in"=w508) -> ("error out"=w509:errorcluster, "Engine Parent Editor Node out"=w505:refnum<class "Engine Parent Editor Node.lvclass">)  [unwired: 7 in]
                  n198 = in-place-dvr #7(w505) -> (w497:errorcluster)  [unwired: 1 out]
                }
                n199 = Merge Errors(w499, w497, w496) -> (w495:errorcluster)
                n200 = Not(x=w495) -> (.not. x?=w494:bool)
              }
            }
            n201 = Compound Arithmetic op=OR(w483, w491) -> (w489:bool)
          }
          event Value Change {
            n202 = event-data() -> ()  [unwired: 1 in, 1 out]
            n203 = Generate User Event(user event=w512, event data cluster=FALSE ("event data")) -> (error out=w510:errorcluster)  [unwired: 2 in, 1 out]
          }
        }
        n204 = case shown="False" w66 {
          tunnel: [w79 w81] -> w65
          tunnel: w64 -> [w80 w81]
          tunnel: w63 -> [w78 _]
          frame False {
            n205 = property on="Property Node" class="Enum (strict)"(reference=w78, error in=w80, "Position"=T10 {"Left"=-1000, "Top"=-1000}) -> (error out=w79:errorcluster)  [unwired: 1 out]
          }
          frame True {
          }
        }
        n206 = case shown="Error" w65 {
          selector: w65 -> [w82 w84]
          tunnel: [w82 errorcluster {"status"=FALSE, "code"=0, "source"=""} ("error IO")] -> w70
          frame No Error {
          }
          frame Error {
            # "#err improve"
            n207 = call <vilib>:"Simple Error Handler.vi"("error in (no error)"=w84) -> ()  [unwired: 4 in, 5 out]
          }
        }
      }
      n208 = case shown="True" w43 {
        tunnel: w42 -> [_ w56]
        tunnel: w41 -> [_ w55]
        frame False {
        }
        frame True {
          n209 = Generate User Event(user event=w56, event data cluster=w55) -> ()  [unwired: 2 in, 2 out]
        }
      }
    }
    frame Error {
    }
  }
  n210 = Unregister For Events(event registration refnum=w37, error in=w36) -> ()  [unwired: 1 out]
